vi "Image Acquistion Main Pxpose.vi"(6 "lpszRefPath":string, 7 "nWindowTime":i32, 8 "error in (no error)":errorcluster, 9 "nMode":u32, 10 "pImage":u16, 11 "nSensorIP":u32) -> (0 "error out":errorcluster, 2 "pImage out":u16, 3 "function return":i32, 4 "lpszRefPath out":string)   [LabVIEW 2017, in "imgAcquisiotn.lvlib"]
doc: "DLLFunction int __stdcall ImageCapImageAcquistionMainPxpose(unsigned int nSensorIP, unsigned short* pImage, unsigned int nMode, int nWindowTime, LPCTSTR lpszRefPath);"
uses:
  imgAcquisiotn.lvlib
  lib/ImageCaptureDLL.dll
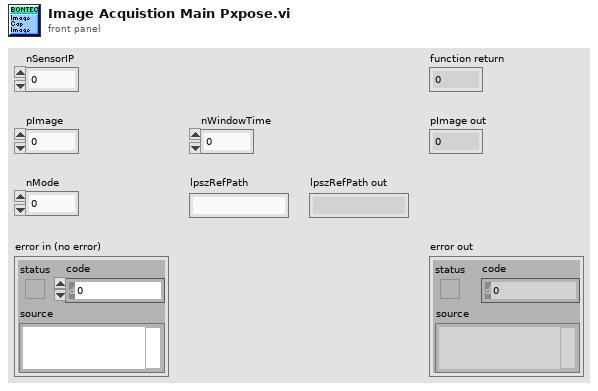
[diagram p1: front panel]
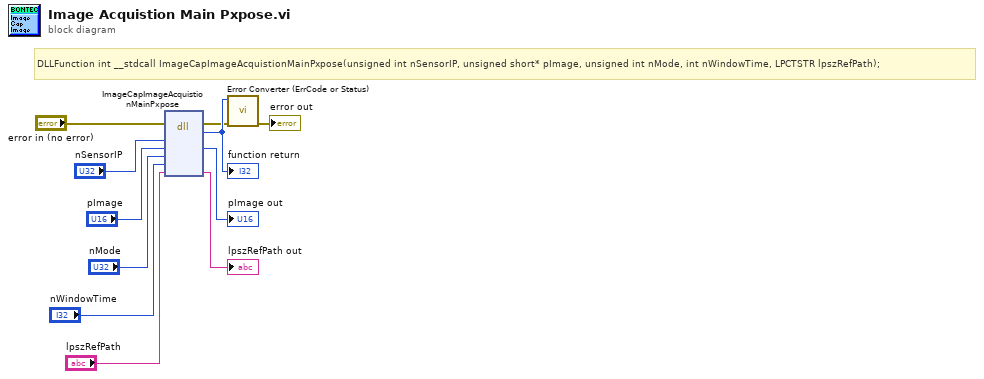
[diagram p0: block diagram]
diagram:
  # "DLLFunction int __stdcall ImageCapImageAcquistionMainPxpose(unsigned int nSensorIP, unsigned short* pImage, unsigned int nMode, int nWindowTime, LPCTSTR lpszRefPath);"
  n1 = dll-call lib="F:/BonTechFlatPanelLVDriver/lib/ImageCaptureDLL.*" fn="ImageCapImageAcquistionMainPxpose"(error in="error in (no error)", "nSensorIP"="nSensorIP", "pImage"="pImage", "nMode"="nMode", "nWindowTime"="nWindowTime", "lpszRefPath"="lpszRefPath") -> (error out=w2:errorcluster, w11:i32, "pImage"=→"pImage out":u16, "lpszRefPath"=→"lpszRefPath out":string)  [unwired: 5 in, 1 out]
  "function return" <- w11
  n2 = call "Error Converter (ErrCode or Status).vi"("error in (no error)"=w2, "error code"=w11) -> ("error out"=→"error out":errorcluster)  [unwired: 9 in]
